vi "Launch Room Service Monitor.vi"(0 "Hotel Management Tool Model in":refnum<class "Hotel Management Tool Model.lvclass">, 11 "error in (no error)":errorcluster) -> (4 "Hotel Management Tool Model out":refnum<class "Hotel Management Tool Model.lvclass">, 15 "error out":errorcluster)   [LabVIEW 2023, in "Hotel Management Tool Model.lvlib" / "Hotel Management Tool Model.lvclass"]
uses:
  Hotel Management Tool Model.lvclass
  Hotel Management Tool Model.lvclass/Hotel Management Tool Model.ctl
  <vilib>/ActorFramework/Actor/Actor.lvclass
  Room Service Monitor Model/Room Service Monitor Model/Room Service Monitor Model.lvclass
  C:/Users/bhaghyaraj/Trainings/NI Actor Framework/SDLC/Model Base/Model Base/Model Base.lvclass
  C:/Program Files/National Instruments/LabVIEW 2023/vi.lib/ActorFramework/Actor/Actor.lvclass
  C:/Users/bhaghyaraj/Trainings/NI Actor Framework/SDLC/Interfaces/Model Base/Incoming Model Base Interface.lvclass
  C:/Users/bhaghyaraj/Trainings/NI Actor Framework/SDLC/Room Service Monitor Model/Room Service Monitor Model/Room Service Monitor Model.lvclass
  C:/Users/bhaghyaraj/Trainings/NI Actor Framework/SDLC/Hotel Management Tool Model/Hotel Management Tool Model/Hotel Management Tool Model.lvclass
  C:/Users/bhaghyaraj/Trainings/NI Actor Framework/SDLC/Interfaces/Hotel Management Tool Model/Incoming Hotel Management Tool Model Interface.lvclass
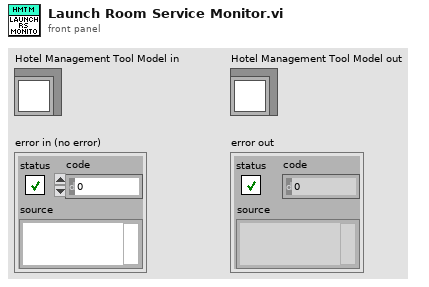
[diagram p1: front panel]
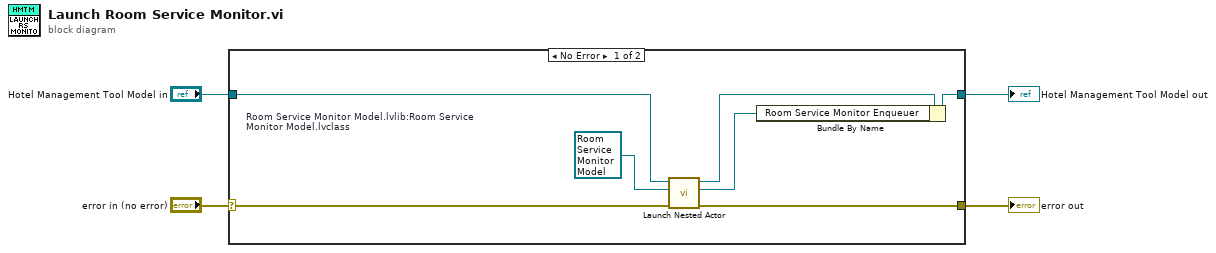
[diagram p0: block diagram]
diagram:
  n1 = case shown="No Error" "error in (no error)" {
    selector: "error in (no error)" -> [w11 w13]
    tunnel: [w10 w13] -> w3
    tunnel: [w7 w12] -> w1
    tunnel: "Hotel Management Tool Model in" -> [w9 w12]
    frame No Error {
      w5 = refnum<class "Room Service Monitor Model.lvclass"> refnum  # Room Service Monitor Model.lvlib:Room Service Monitor Model.lvclass
      n2 = call <vilib>:"Launch Nested Actor.vi"("error in (no error)"=w11, "Nested Actor"=w5, "Caller Actor in"=w9) -> ("error out"=w10:errorcluster, "Nested Actor's Enqueuer"=w6:refnum<class "Message Enqueuer.lvclass">, "Caller Actor out"=w8:refnum<class "Hotel Management Tool Model.lvclass">)  [unwired: 6 in]
      n3 = Bundle By Name(cluster=w8, "Room Service Monitor Enqueuer"=w6) -> (w7:refnum<class "Hotel Management Tool Model.lvclass">)
    }
    frame Error {
    }
  }
  "error out" <- w3
  "Hotel Management Tool Model out" <- w1
